vi "ex_Handle Radio Buttons.vi"(5 "Reinitialize":bool, 6 "Inverted Boolean Control":string, 7 "Boolean Control":string, 8 "error in (no error)":errorcluster, 9 "Numeric Control":string, 10 "Radio Buttons":string[](array[string]), 11 "VI refnum":refnum<vi>) -> (0 "error out":errorcluster, 1 "Radio Button Ctrl Refs":refnum<vi>[](array[refnum]), 2 "Selected Button":u32, 3 "Changed?":bool)   [LabVIEW 2020]
doc: "Makes an array of buttons act like a set of radio buttons and returns a Boolean indicating if the radio buttons have changed state an integer indicating which of the radio buttons is pressed.\n\nYou input the VI refnum for the VI panel containing the radio buttons and an array of the button label names. You also input the label for a numeric control, Boolean control, or inverted Boolean control that you want to be associated with the result of the radio buttons. On the first time it is run, it itinitializes the buttons based on the value of the inputs. This also happens when the Reinitiaize boolean is true."
panel:
  in  "Could not find radio button:":string="Radio button: "
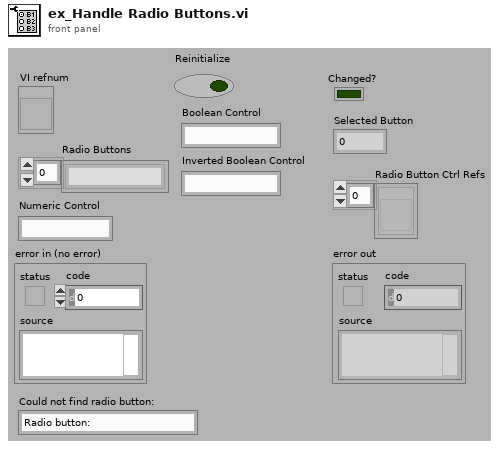
[diagram p1: front panel]
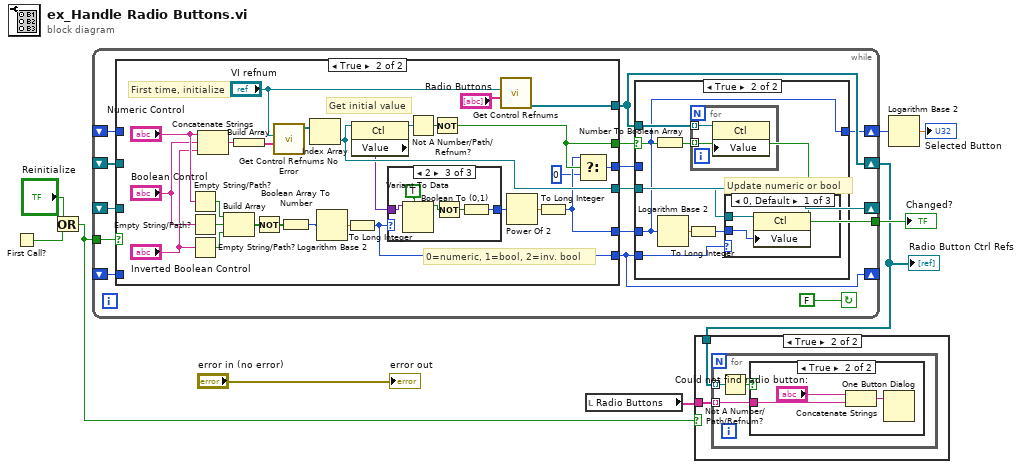
[diagram p0: block diagram]
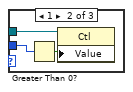
[diagram p5: hidden frame]
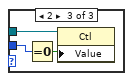
[diagram p6: hidden frame]
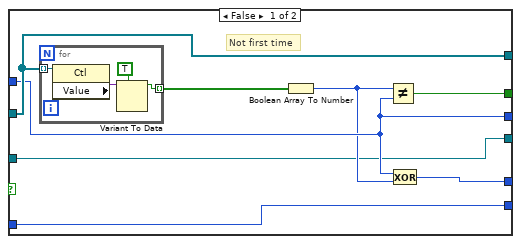
[diagram p7: hidden frame]
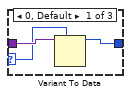
[diagram p8: hidden frame]
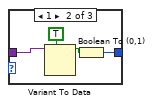
[diagram p9: hidden frame]
diagram:
  n1 = First Call?() -> (First Call?: T/F=w2:bool)
  n2 = Or(x="Reinitialize", y=w2) -> (x .or. y?=w1:bool)
  n3 = while {
    shift-right: [w14] -> w4
    shift-left: _ -> [w20]
    tunnel: w1 -> [w21]
    shift-right: [w11] -> w8
    shift-left: _ -> [w19]
    shift-right: [w16] -> _
    shift-left: _ -> [w18]
    tunnel: [w10] -> w7
    shift-right: [w15] -> _
    shift-left: _ -> [w17]
    stop <- FALSE continue-if-true
    n4 = case shown="True" w21 {
      tunnel: [w45 w78] -> w14
      tunnel: w20 -> [w45 _]
      tunnel: w19 -> [w44 _]
      tunnel: [w47 w55] -> w10
      tunnel: [w41 w70] -> w16
      tunnel: w18 -> [w41 _]
      tunnel: [w46 w62] -> w15
      tunnel: w17 -> [w46 _]
      tunnel: [w42 w54] -> w12
      tunnel: [w44 w56] -> w13
      frame False {
        # "Not first time"
        n5 = for {
          tunnel: w45 -> [w52] mode=indexing
          tunnel: [w49] -> w48 mode=indexing
          n6 = property class="Ctl"(reference=w52) -> ("Value"=w51:variant)  [unwired: 1 in, 2 out]
          n7 = Variant To Data(type=TRUE, Variant=w51) -> (data=w49:bool)  [unwired: 1 in, 1 out]
        }
        n8 = Boolean Array To Number(Boolean array=w48) -> (number=w43:u32)
        n9 = Not Equal?(x=w43, y=w44) -> (x != y?=w47:bool)
        n10 = Exclusive Or(1:w43, 2:w44) -> (0:w42:u32)
      }
      frame True {
        # "Get initial value"
        # "0=numeric, 1=bool, 2=inv. bool"
        # "First time, initialize"
        n11 = Empty String/Path?(string/path="Numeric Control") -> (empty?=w65:bool)
        n12 = Empty String/Path?(string/path="Boolean Control") -> (empty?=w77:bool)
        n13 = Empty String/Path?(string/path="Inverted Boolean Control") -> (empty?=w76:bool)
        n14 = Concatenate Strings("Numeric Control", "Boolean Control", "Inverted Boolean Control") -> (w67:string)
        n15 = Build Array(w65, w77, w76) -> (w75:bool[])
        n16 = Build Array(w67) -> (w66:string[])
        n17 = Not(x=w75) -> (.not. x?=w59:bool[])
        n18 = call <vilib>:"Get Control Refnums No Error.vi"("Names"=w66, "viref Block"="VI refnum") -> ("Refs Output"=w68:refnum<vi>[])  [unwired: 7 in, 2 out]
        n19 = Boolean Array To Number(Boolean array=w59) -> (number=w74:u32)
        n20 = Index Array(array=w68) -> (element=w70:refnum<vi>)  [unwired: 1 in]
        n21 = Logarithm Base 2(1:w74) -> (0:w69:dbl)
        n22 = To Long Integer(number=w69) -> (32bit integer=w62:i32)
        n23 = property class="Ctl"(reference=w70) -> (reference out=w58:refnum<vi>, "Value"=w63:variant)  [unwired: 1 in, 1 out]
        n24 = case shown="2" w62 {
          selector: w62 -> [w81 _ _]
          tunnel: w63 -> [w82 w86 w91]
          tunnel: [w80 w84 w90] -> w61
          frame 0, Default {
            n25 = Variant To Data(type=w81, Variant=w82) -> (data=w80:i32)  [unwired: 1 in, 1 out]
          }
          frame 1 {
            n26 = Variant To Data(type=TRUE, Variant=w86) -> (data=w85:bool)  [unwired: 1 in, 1 out]
            n27 = Boolean To (0,1)(Boolean=w85) -> (0, 1=w84:i16)
          }
          frame 2 {
            n28 = Variant To Data(type=TRUE, Variant=w91) -> (data=w89:bool)  [unwired: 1 in, 1 out]
            n29 = Not(x=w89) -> (.not. x?=w88:bool)
            n30 = Boolean To (0,1)(Boolean=w88) -> (0, 1=w90:i16)
          }
        }
        n31 = Not A Number/Path/Refnum?(number/path/refnum=w58) -> (NaN/Path/Refnum?=w57:bool)
        n32 = Not(x=w57) -> (.not. x?=w55:bool)
        n33 = call <vilib>:"Get Control Refnums.vi"("Names"="Radio Buttons", "viref Block"="VI refnum") -> ("Refs Output"=w78:refnum<vi>[])  [unwired: 7 in, 2 out]
        n34 = Power Of 2(x=w61) -> (2^x=w60:dbl)
        n35 = To Long Integer(number=w60) -> (32bit integer=w54:i32)
        n36 = Select(t=w54, s=w55, f=0) -> (s? t:f=w56:i32)
      }
    }
    n37 = case shown="True" w10 {
      tunnel: w14 -> [_ w29]
      tunnel: w15 -> [_ w26]
      tunnel: w12 -> [_ w25]
      tunnel: w16 -> [_ w24]
      tunnel: w13 -> [w23 _]
      tunnel: [w23 w25] -> w11
      frame False {
        # "No changes"
      }
      frame True {
        # "Update numeric or bool"
        n38 = Number To Boolean Array(number=w25) -> (Boolean array=w30:bool[])
        n39 = Logarithm Base 2(1:w25) -> (0:w28:dbl)
        n40 = To Long Integer(number=w28) -> (32bit integer=w27:i32)
        n41 = for {
          tunnel: w30 -> [w39] mode=indexing
          tunnel: w29 -> [w40] mode=indexing
          n42 = property class="Ctl"(reference=w40, "Value"=w39) -> ()  [unwired: 1 in, 2 out]
        }
        n43 = case shown="0, Default" w26 {
          tunnel: w27 -> [w31 w35 w37]
          tunnel: w24 -> [w32 w33 w38]
          frame 0, Default {
            n44 = property class="Ctl"(reference=w32, "Value"=w31) -> ()  [unwired: 1 in, 2 out]
          }
          frame 1 {
            n45 = Greater Than 0?(x=w35) -> (x > 0?=w34:bool)
            n46 = property class="Ctl"(reference=w33, "Value"=w34) -> ()  [unwired: 1 in, 2 out]
          }
          frame 2 {
            n47 = Equal To 0?(x=w37) -> (x = 0?=w36:bool)
            n48 = property class="Ctl"(reference=w38, "Value"=w36) -> ()  [unwired: 1 in, 2 out]
          }
        }
      }
    }
  }
  "Changed?" <- w7
  "Radio Button Ctrl Refs" <- w4
  n49 = local read "Radio Buttons"() -> (w6:string[])
  n50 = case shown="True" w1 {
    tunnel: w4 -> [_ w93]
    tunnel: w6 -> [_ w92]
    frame False {
    }
    frame True {
      n51 = for {
        tunnel: w93 -> [w96] mode=indexing
        tunnel: w92 -> [w94] mode=indexing
        n52 = Not A Number/Path/Refnum?(number/path/refnum=w96) -> (NaN/Path/Refnum?=w95:bool)
        n53 = case shown="True" w95 {
          tunnel: w94 -> [_ w99]
          frame False {
          }
          frame True {
            n54 = Concatenate Strings("Could not find radio button:", w99) -> (w97:string)
            n55 = One Button Dialog(message=w97) -> ()  [unwired: 1 in, 1 out]
          }
        }
      }
    }
  }
  n56 = Logarithm Base 2(1:w8) -> (0:→"Selected Button":dbl)
  "error out" <- "error in (no error)"
